vi "Close Device.vi"(8 "error in (no error)":errorcluster, 11 "LightBox in":refnum<class "LightBox.lvclass">) -> (0 "error out":errorcluster, 3 "LightBox out":refnum<class "LightBox.lvclass">)   [LabVIEW 2016, in "LightBox.lvclass"]
uses:
  LightBox.lvclass
  LightBox.lvclass/LightBox.ctl
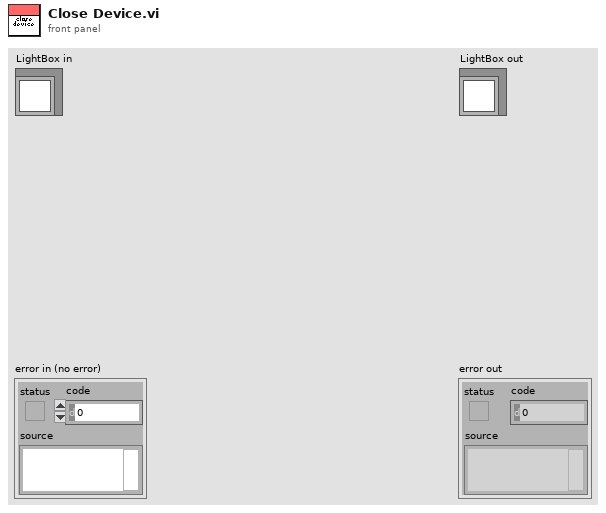
[diagram p1: front panel]
types:
  T1 = typedef "Platinum_MB_SerHandle.ctl" = cluster{"VISAResourceName":string, "Mode":T2, "Timeout":u32, "FlowControl":T3, "Parity":T4, "BaudRate":u32, "SlaveAddress":u8}
  T2 = typedef "Platinum_MB_serMode.ctl" = enum16{"RTU", "ASCII"}
  T3 = typedef "Platinum_MB_serFlowControl.ctl" = enum16{"None", "XON_XOFF", "RTS_CTS", "XON_XOFF_and_RTS_CTS", "DTR_DSR", "XON_XOFF_and_DTR_DSR"}
  T4 = typedef "Platinum_MB_serParity.ctl" = enum16{"None", "Odd", "Even", "Mark", "Space"}
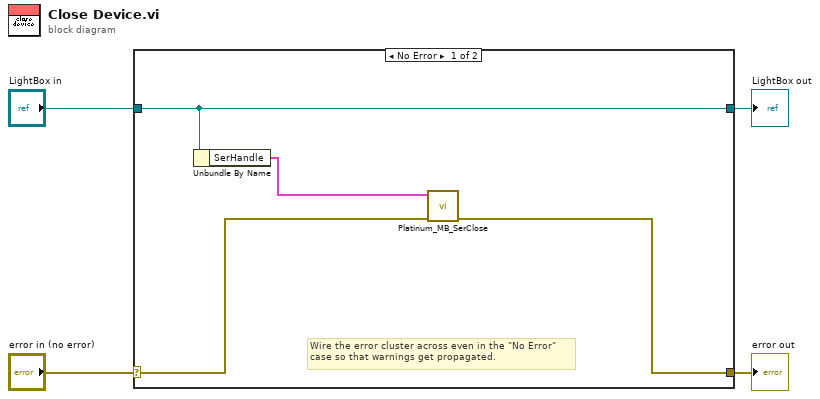
[diagram p0: block diagram]
diagram:
  n1 = case shown="No Error" "error in (no error)" {
    selector: "error in (no error)" -> [w8 w10]
    tunnel: [w7 w10] -> w3
    tunnel: [w6 w9] -> w1
    tunnel: "LightBox in" -> [w6 w9]
    frame No Error {
      # "Wire the error cluster across even in the \"No Error\"\ncase so that warnings get propagated."
      n2 = Unbundle By Name(w6) -> ("SerHandle"=w5:T1)
      n3 = call "Platinum_MB_SerClose.vi"("error in (no error)"=w8, "SerHandle"=w5) -> ("error out"=w7:errorcluster)  [unwired: 9 in]
    }
    frame Error {
    }
  }
  "error out" <- w3
  "LightBox out" <- w1
